vi "MatchCameraImages.vi"(1 "R_TargetArray":T1(array[cluster]), 2 "L_TargetArray":T1(array[cluster])) -> (0 "TargetMatch":T2(array[cluster]))   [LabVIEW 2011]
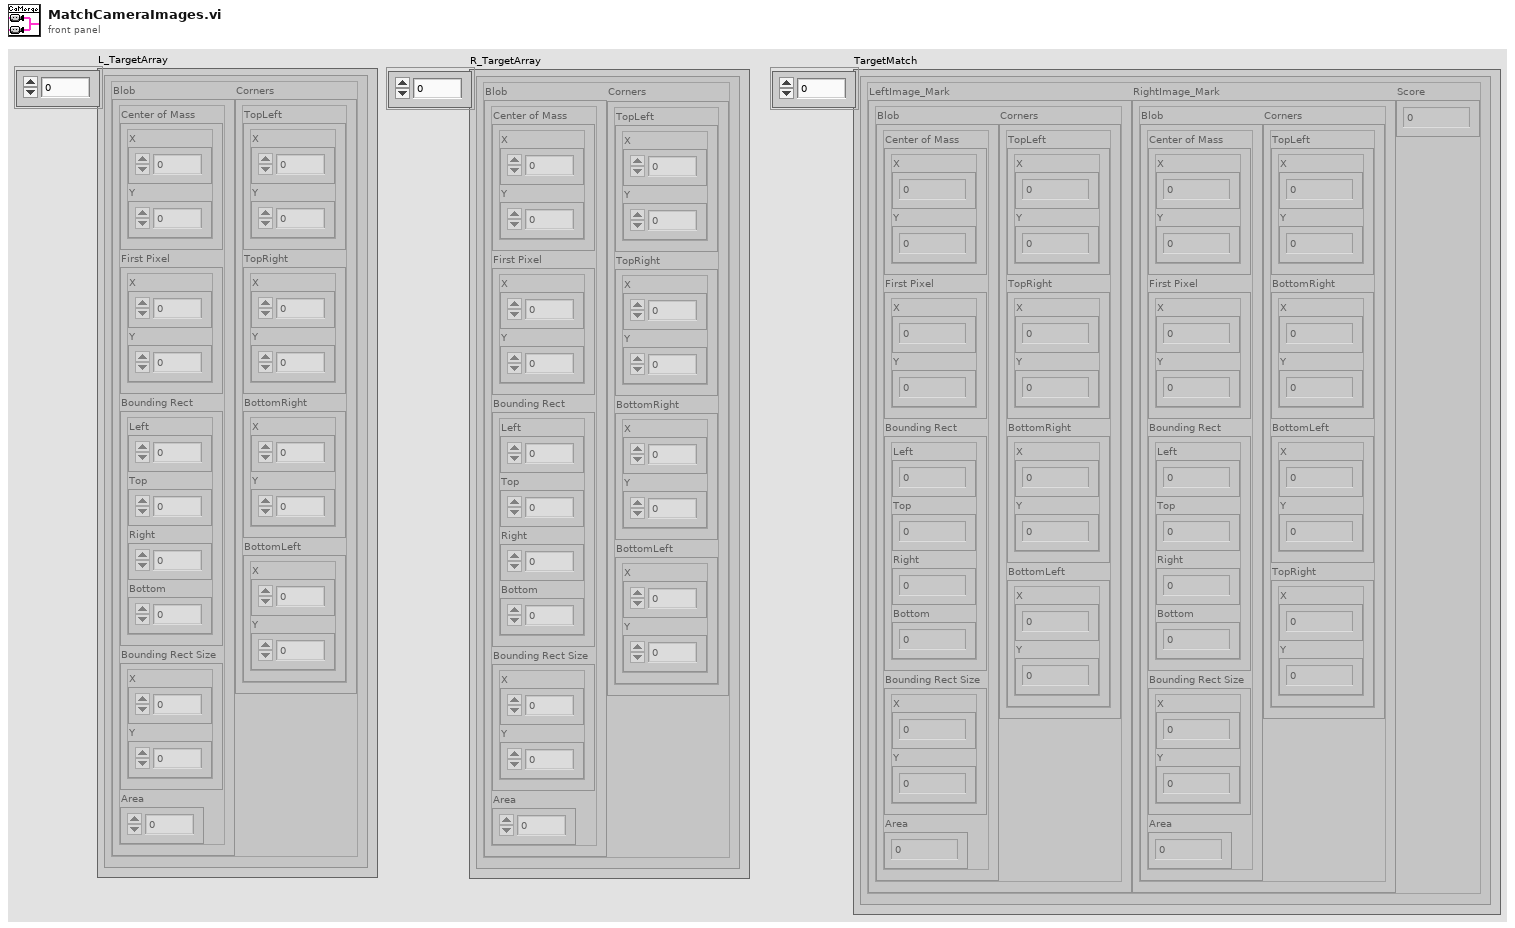
[diagram p1: front panel]
types:
  T1 = cluster{"Blob":cluster{"Center of Mass":cluster{"X":dbl, "Y":dbl}, "First Pixel":cluster{"X":dbl, "Y":dbl}, "Bounding Rect":cluster{"Left":dbl, "Top":dbl, "Right":dbl, "Bottom":dbl}, "Bounding Rect Size":cluster{"X":dbl, "Y":dbl}, "Area":dbl}, "Corners":cluster{"TopLeft":cluster{"X":dbl, "Y":dbl}, "TopRight":cluster{"X":dbl, "Y":dbl}, "BottomRight":cluster{"X":dbl, "Y":dbl}, "BottomLeft":cluster{"X":dbl, "Y":dbl}}}[]
  T2 = cluster{"LeftImage_Mark":cluster{"Blob":cluster{"Center of Mass":cluster{"X":dbl, "Y":dbl}, "First Pixel":cluster{"X":dbl, "Y":dbl}, "Bounding Rect":cluster{"Left":dbl, "Top":dbl, "Right":dbl, "Bottom":dbl}, "Bounding Rect Size":cluster{"X":dbl, "Y":dbl}, "Area":dbl}, "Corners":cluster{"TopLeft":cluster{"X":dbl, "Y":dbl}, "TopRight":cluster{"X":dbl, "Y":dbl}, "BottomRight":cluster{"X":dbl, "Y":dbl}, "BottomLeft":cluster{"X":dbl, "Y":dbl}}}, "RightImage_Mark":cluster{"Blob":cluster{"Center of Mass":cluster{"X":dbl, "Y":dbl}, "First Pixel":cluster{"X":dbl, "Y":dbl}, "Bounding Rect":cluster{"Left":dbl, "Top":dbl, "Right":dbl, "Bottom":dbl}, "Bounding Rect Size":cluster{"X":dbl, "Y":dbl}, "Area":dbl}, "Corners":cluster{"TopLeft":cluster{"X":dbl, "Y":dbl}, "BottomRight":cluster{"X":dbl, "Y":dbl}, "BottomLeft":cluster{"X":dbl, "Y":dbl}, "TopRight":cluster{"X":dbl, "Y":dbl}}}, "Score":dbl}[]
  T3 = cluster{cluster{"Blob":cluster{"Center of Mass":cluster{"X":dbl, "Y":dbl}, "First Pixel":cluster{"X":dbl, "Y":dbl}, "Bounding Rect":cluster{"Left":dbl, "Top":dbl, "Right":dbl, "Bottom":dbl}, "Bounding Rect Size":cluster{"X":dbl, "Y":dbl}, "Area":dbl}, cluster{"TopLeft":cluster{"X":dbl, "Y":dbl}, "BottomRight":cluster{"X":dbl, "Y":dbl}, "BottomLeft":cluster{"X":dbl, "Y":dbl}, "TopRight":cluster{"X":dbl, "Y":dbl}}}, cluster{"Blob":cluster{"Center of Mass":cluster{"X":dbl, "Y":dbl}, "First Pixel":cluster{"X":dbl, "Y":dbl}, "Bounding Rect":cluster{"Left":dbl, "Top":dbl, "Right":dbl, "Bottom":dbl}, "Bounding Rect Size":cluster{"X":dbl, "Y":dbl}, "Area":dbl}, cluster{"TopLeft":cluster{"X":dbl, "Y":dbl}, "BottomRight":cluster{"X":dbl, "Y":dbl}, "BottomLeft":cluster{"X":dbl, "Y":dbl}, "TopRight":cluster{"X":dbl, "Y":dbl}}}, dbl}[]
  T4 = cluster{"Blob":cluster{"Center of Mass":cluster{"X":dbl, "Y":dbl}, "First Pixel":cluster{"X":dbl, "Y":dbl}, "Bounding Rect":cluster{"Left":dbl, "Top":dbl, "Right":dbl, "Bottom":dbl}, "Bounding Rect Size":cluster{"X":dbl, "Y":dbl}, "Area":dbl}, cluster{"TopLeft":cluster{"X":dbl, "Y":dbl}, "BottomRight":cluster{"X":dbl, "Y":dbl}, "BottomLeft":cluster{"X":dbl, "Y":dbl}, "TopRight":cluster{"X":dbl, "Y":dbl}}}
  T5 = cluster{"Center of Mass":cluster{"X":dbl, "Y":dbl}, "First Pixel":cluster{"X":dbl, "Y":dbl}, "Bounding Rect":cluster{"Left":dbl, "Top":dbl, "Right":dbl, "Bottom":dbl}, "Bounding Rect Size":cluster{"X":dbl, "Y":dbl}, "Area":dbl}
  T6 = cluster{"Left":dbl, "Top":dbl, "Right":dbl, "Bottom":dbl}
  T7 = cluster{"Blob":cluster{"Center of Mass":cluster{"X":dbl, "Y":dbl}, "First Pixel":cluster{"X":dbl, "Y":dbl}, "Bounding Rect":cluster{"Left":dbl, "Top":dbl, "Right":dbl, "Bottom":dbl}, "Bounding Rect Size":cluster{"X":dbl, "Y":dbl}, "Area":dbl}, "Corners":cluster{"TopLeft":cluster{"X":dbl, "Y":dbl}, "BottomRight":cluster{"X":dbl, "Y":dbl}, "BottomLeft":cluster{"X":dbl, "Y":dbl}, "TopRight":cluster{"X":dbl, "Y":dbl}}}
  T8 = cluster{"Cluster":cluster{"Blob":cluster{"Center of Mass":cluster{"X":dbl, "Y":dbl}, "First Pixel":cluster{"X":dbl, "Y":dbl}, "Bounding Rect":cluster{"Left":dbl, "Top":dbl, "Right":dbl, "Bottom":dbl}, "Bounding Rect Size":cluster{"X":dbl, "Y":dbl}, "Area":dbl}, "Corners":cluster{"TopLeft":cluster{"X":dbl, "Y":dbl}, "TopRight":cluster{"X":dbl, "Y":dbl}, "BottomRight":cluster{"X":dbl, "Y":dbl}, "BottomLeft":cluster{"X":dbl, "Y":dbl}}}, cluster{"Blob":cluster{"Center of Mass":cluster{"X":dbl, "Y":dbl}, "First Pixel":cluster{"X":dbl, "Y":dbl}, "Bounding Rect":cluster{"Left":dbl, "Top":dbl, "Right":dbl, "Bottom":dbl}, "Bounding Rect Size":cluster{"X":dbl, "Y":dbl}, "Area":dbl}, cluster{"TopLeft":cluster{"X":dbl, "Y":dbl}, "BottomRight":cluster{"X":dbl, "Y":dbl}, "BottomLeft":cluster{"X":dbl, "Y":dbl}, "TopRight":cluster{"X":dbl, "Y":dbl}}}, dbl}
  T9 = cluster{"Cluster":cluster{"Blob":cluster{"Center of Mass":cluster{"X":dbl, "Y":dbl}, "First Pixel":cluster{"X":dbl, "Y":dbl}, "Bounding Rect":cluster{"Left":dbl, "Top":dbl, "Right":dbl, "Bottom":dbl}, "Bounding Rect Size":cluster{"X":dbl, "Y":dbl}, "Area":dbl}, "Corners":cluster{"TopLeft":cluster{"X":dbl, "Y":dbl}, "TopRight":cluster{"X":dbl, "Y":dbl}, "BottomRight":cluster{"X":dbl, "Y":dbl}, "BottomLeft":cluster{"X":dbl, "Y":dbl}}}, cluster{"Blob":cluster{"Center of Mass":cluster{"X":dbl, "Y":dbl}, "First Pixel":cluster{"X":dbl, "Y":dbl}, "Bounding Rect":cluster{"Left":dbl, "Top":dbl, "Right":dbl, "Bottom":dbl}, "Bounding Rect Size":cluster{"X":dbl, "Y":dbl}, "Area":dbl}, cluster{"TopLeft":cluster{"X":dbl, "Y":dbl}, "BottomRight":cluster{"X":dbl, "Y":dbl}, "BottomLeft":cluster{"X":dbl, "Y":dbl}, "TopRight":cluster{"X":dbl, "Y":dbl}}}, dbl}[]
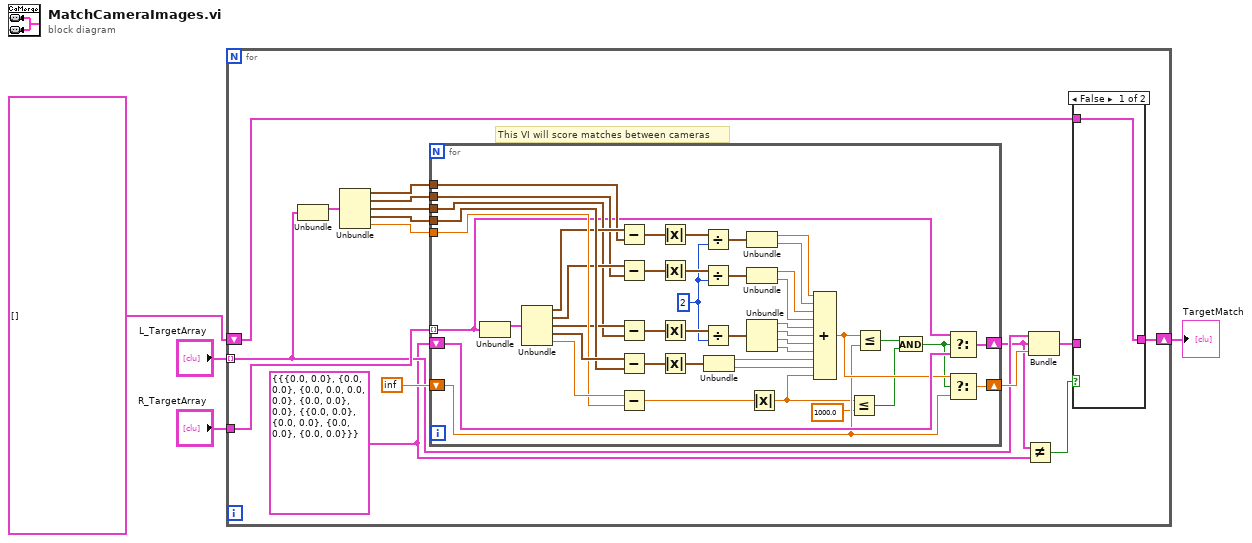
[diagram p0: block diagram]
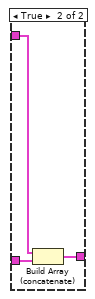
[diagram p2: hidden frame]
diagram:
  n1 = for {
    tunnel: "L_TargetArray" -> [w8] mode=indexing
    tunnel: "R_TargetArray" -> [w20]
    shift-right: [w16] -> w1
    shift-left: T3 [] -> [w15]
    w6 = T4 {"Blob"={"Center of Mass"={"X"=0.0, "Y"=0.0}, "First Pixel"={"X"=0.0, "Y"=0.0}, "Bounding Rect"={"Left"=0.0, "Top"=0.0, "Right"=0.0, "Bottom"=0.0}, "Bounding Rect Size"={"X"=0.0, "Y"=0.0}, "Area"=0.0}, {"TopLeft"={"X"=0.0, "Y"=0.0}, "BottomRight"={"X"=0.0, "Y"=0.0}, "BottomLeft"={"X"=0.0, "Y"=0.0}, "TopRight"={"X"=0.0, "Y"=0.0}}}
    # "This VI will score matches between cameras"
    n2 = Unbundle(w8) -> ("Blob"=w9:T5)  [unwired: 1 out]
    n3 = Unbundle(w9) -> ("Center of Mass"=w14:cluster{"X":dbl, "Y":dbl}, "First Pixel"=w13:cluster{"X":dbl, "Y":dbl}, "Bounding Rect"=w12:T6, "Bounding Rect Size"=w19:cluster{"X":dbl, "Y":dbl}, "Area"=w18:dbl)
    n4 = for {
      tunnel: w20 -> [w30] mode=indexing
      tunnel: w18 -> [w67]
      tunnel: w19 -> [w65]
      shift-right: [w36] -> w7
      shift-left: w6 -> [w40]
      tunnel: w14 -> [w60]
      tunnel: w13 -> [w59]
      tunnel: w12 -> [w58]
      shift-right: [w37] -> w10
      shift-left: inf -> [w38]
      w32 = 2
      n5 = Unbundle(w30) -> ("Blob"=w31:T5)  [unwired: 1 out]
      n6 = Unbundle(w31) -> ("Center of Mass"=w63:cluster{"X":dbl, "Y":dbl}, "First Pixel"=w62:cluster{"X":dbl, "Y":dbl}, "Bounding Rect"=w61:T6, "Bounding Rect Size"=w69:cluster{"X":dbl, "Y":dbl}, "Area"=w68:dbl)
      n7 = Subtract(x=w63, y=w60) -> (x-y=w57:cluster{"X":dbl, "Y":dbl})
      n8 = Subtract(x=w62, y=w59) -> (x-y=w56:cluster{"X":dbl, "Y":dbl})
      n9 = Subtract(x=w61, y=w58) -> (x-y=w55:T6)
      n10 = Subtract(x=w69, y=w65) -> (x-y=w66:cluster{"X":dbl, "Y":dbl})
      n11 = Subtract(x=w68, y=w67) -> (x-y=w64:dbl)
      n12 = Absolute Value(x=w57) -> (abs(x)=w54:cluster{"X":dbl, "Y":dbl})
      n13 = Absolute Value(x=w56) -> (abs(x)=w53:cluster{"X":dbl, "Y":dbl})
      n14 = Absolute Value(x=w55) -> (abs(x)=w52:T6)
      n15 = Absolute Value(x=w66) -> (abs(x)=w43:cluster{"X":dbl, "Y":dbl})
      n16 = Divide(x=w54, y=w32) -> (x/y=w35:cluster{"X":dbl, "Y":dbl})
      n17 = Divide(x=w53, y=w32) -> (x/y=w34:cluster{"X":dbl, "Y":dbl})
      n18 = Divide(x=w52, y=w32) -> (x/y=w33:T6)
      n19 = Unbundle(w43) -> ("X"=w42:dbl, "Y"=w41:dbl)
      n20 = Unbundle(w35) -> ("X"=w51:dbl, "Y"=w50:dbl)
      n21 = Unbundle(w34) -> ("X"=w49:dbl, "Y"=w48:dbl)
      n22 = Unbundle(w33) -> ("Left"=w47:dbl, "Top"=w46:dbl, "Right"=w45:dbl, "Bottom"=w44:dbl)
      n23 = Absolute Value(x=w64) -> (abs(x)=w29:dbl)
      n24 = Compound Arithmetic op=ADD(w51, w50, w49, w48, w47, w46, w45, w44, w42, w41, w29) -> (w39:dbl)
      n25 = Less Or Equal?(x=w29, y=1000.0) -> (x <= y?=w25:bool)
      n26 = Less Or Equal?(x=w39, y=w38) -> (x <= y?=w26:bool)
      n27 = And(x=w26, y=w25) -> (x .and. y?=w27:bool)
      n28 = Select(t=w30, s=w27, f=w40) -> (s? t:f=w36:T7)
      n29 = Select(t=w39, s=w27, f=w38) -> (s? t:f=w37:dbl)
    }
    n30 = Not Equal?(x=w7, y=w6) -> (x != y?=w5:bool)
    n31 = Bundle("Cluster"=w8, w7, w10) -> (w17:T8)  [unwired: 1 in]
    n32 = case shown="False" w5 {
      tunnel: w17 -> [_ w24]
      tunnel: [w21 w23] -> w16
      tunnel: w15 -> [w21 w22]
      frame False {
      }
      frame True {
        n33 = Build Array (concatenate)(w22, w24) -> (w23:T9)
      }
    }
  }
  "TargetMatch" <- w1
